vi "Get Bus Status Channel Names.vi"() -> (2 "bus status loads":string[](array[string]), 3 "bus status counts":string[](array[string]))   [LabVIEW 2020, in "AIM MIL-STD-1553 Scripting.lvlib"]
uses:
  AIM MIL-STD-1553 Scripting.lvlib
  Constants.vi
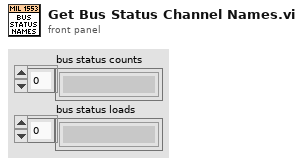
[diagram p1: front panel]
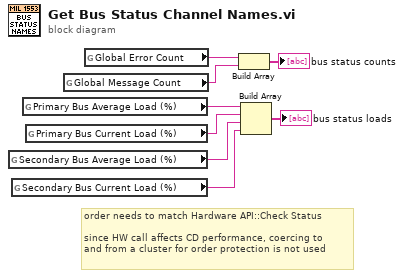
[diagram p0: block diagram]
diagram:
  # "order needs to match Hardware API::Check Status\n\nsince HW call affects CD performance, coercing to \nand from a cluster for order protection is not used"
  n1 = global read "Constants.vi" "Secondary Bus Average Load (%)"() -> (w6:string)
  n2 = global read "Constants.vi" "Secondary Bus Current Load (%)"() -> (w5:string)
  n3 = global read "Constants.vi" "Primary Bus Average Load (%)"() -> (w8:string)
  n4 = global read "Constants.vi" "Primary Bus Current Load (%)"() -> (w7:string)
  n5 = global read "Constants.vi" "Global Message Count"() -> (w4:string)
  n6 = global read "Constants.vi" "Global Error Count"() -> (w3:string)
  n7 = Build Array(w3, w4) -> (→"bus status counts":string[])
  n8 = Build Array(w8, w7, w6, w5) -> (→"bus status loads":string[])
